vi "Save Images Tool.vi"(8 "Error In":errorcluster) -> (0 "Error Out":errorcluster)   [LabVIEW 2011]
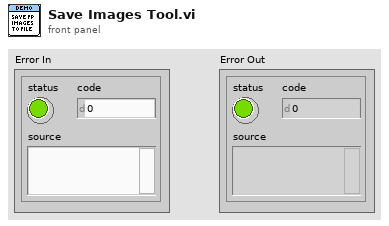
[diagram p1: front panel]
types:
  T1 = typedef "imagedata.ctl" = cluster{"image type":i32, "image depth":i32, "image":u8[], "mask":u8[], "colors":u32[], "Rectangle":cluster{"left":i16, "top":i16, "right":i16, "bottom":i16}}
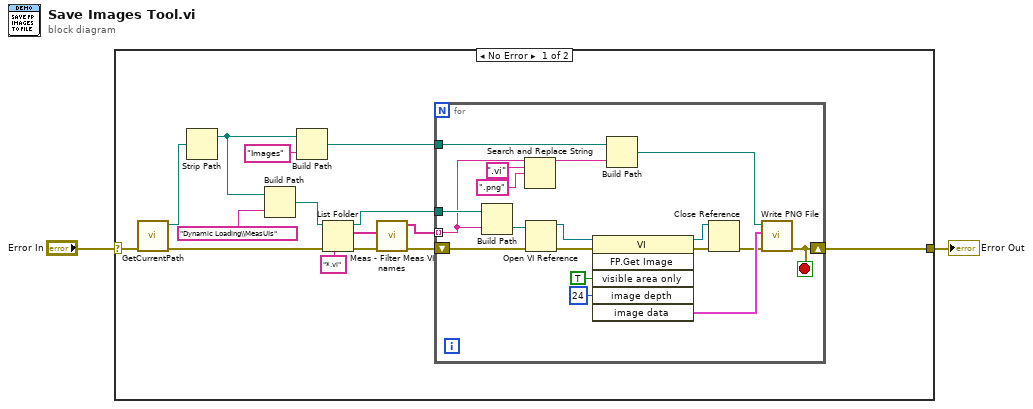
[diagram p0: block diagram]
diagram:
  n1 = case shown="No Error" "Error In" {
    selector: "Error In" -> [w10 w36]
    tunnel: [w7 w36] -> w2
    frame No Error {
      n2 = call "GetCurrentPath.vi"("Error In"=w10) -> ("Error Out"=w9:errorcluster, "Current VI Path Out"=w11:path)  [unwired: 9 in]
      n3 = Strip Path(path=w11) -> (stripped path=w12:path)  [unwired: 1 out]
      n4 = Build Path(base path=w12, name or relative path="Dynamic Loading\\MeasUIs") -> (appended path=w16:path)
      n5 = Build Path(base path=w12, name or relative path="Images") -> (appended path=w8:path)
      n6 = List Folder(path=w16, pattern="*.vi", error in=w9) -> (path out=w14:path, filenames=w4:string[], error out=w6:errorcluster)  [unwired: 1 in, 1 out]
      n7 = call "Meas - Filter Meas VI names.vi"("error in"=w6, "filenames In"=w4) -> ("Error Out"=w5:errorcluster, "Meas VIs Out"=w3:string[])  [unwired: 8 in]
      n8 = for {
        tunnel: w3 -> [w29] mode=indexing
        tunnel: w14 -> [w35]
        shift-right: [w23] -> w7
        shift-left: w5 -> [w32]
        tunnel: w8 -> [w25]
        stop <- w23 stop-if-true
        n9 = Build Path(base path=w35, name or relative path=w29) -> (appended path=w31:path)
        n10 = Search and Replace String(input string=w29, search string=".vi", replace string=".png" ("search string")) -> (result string=w26:string)  [unwired: 5 in, 3 out]
        n11 = Open VI Reference(vi path=w31, error in (no error)=w32) -> (vi reference=w22:refnum<vi>, error out=w30:errorcluster)  [unwired: 4 in]
        n12 = invoke class="VI" method="FP.Get Image"(reference=w22, error in=w30, "visible area only"=TRUE ("Visible Area Only"), "image depth"=24 ("Image Depth")) -> (reference out=w19:refnum<vi>, error out=w20:errorcluster, "image data"=w24:T1)  [unwired: 2 in, 3 out]
        n13 = Build Path(base path=w25, name or relative path=w26) -> (appended path=w18:path)
        n14 = Close Reference(reference=w19, error in (no error)=w20) -> (error out=w21:errorcluster)
        n15 = call <vilib>:"Write PNG File.vi"("error in (no error)"=w21, "image data"=w24, "path to PNG file"=w18) -> ("error out"=w23:errorcluster)  [unwired: 7 in, 1 out]
      }
    }
    frame Error {
    }
  }
  "Error Out" <- w2
